vi "Hindbrain Main.vi"(8 "Boat Type":T1, 9 "XBee Serial Port":refnum<visa-resource-name>="LPT1", 11 "NotifierReff":T5) -> ()   [LabVIEW 2013]
doc: "Place to hold all the hindbrain code."
uses:
  Data/TypeDefs/Notifiers.ctl
  Data/TypeDefs/UTM Location.ctl
  Data/TypeDefs/Sail Set Suggestions.ctl
  Data/TypeDefs/Rudder Set Suggestions.ctl
  Data/TypeDefs/OverrideInformation.ctl
  Data/TypeDefs/OverrideMode.ctl
  Data/TypeDefs/MotorSetup.ctl
  Data/TypeDefs/DynamixelSetupInfo.ctl
  Data/TypeDefs/AirmarStatus.ctl
  Data/TypeDefs/HardwareOnline.ctl
  Data/TypeDefs/DynamixelCycleTracker.ctl
  Data/TypeDefs/RC Input Values.ctl
  Classes/Waypoint/Waypoint.lvclass
  Data/TypeDefs/BoatType.ctl
  <vilib>/myRIO/Common/Instrument Driver Framework/myRIO v1.0/UART/vis/myRIO v1.0 Close UART.vi
  <vilib>/myRIO/Common/Instrument Driver Framework/Utilities/vis/FPGA Ref Manager.vi
  <vilib>/myRIO/Common/Instrument Driver Framework/myRIO v1.0/myRIO v1.0 Reset FPGA.vi
  <vilib>/myRIO/Instrument Drivers/Utilities/Utilities.lvlib
  <instrlib>/Dynamixel Motor/Dynamixel Motor.lvlib
panel:
  in  "Tab Control":T2(tab)
  out "Write loop\ncounter":i32
  out "Commanded rudder value":T3 min=-0.95 max=0.95 scale=1.0..-1.0
  out "Commanded sail value":dbl
  out "Dynamixel\nPositions (deg)":dbl[](array[numeric])
  in  "Read actions per\nwrite action":i32=4
  out "Think Counter":i32
  out "Think Heartbeat":bool
  out "Sense Counter":i32
  out "Sense Heartbeat":bool
  out "Act Heartbeat":bool
  out "Read loop counter":i32
  out "Updated Dynamixel Cycles":T4
  in  "Motors Enabled":bool[](array[boolean])=[TRUE, TRUE, TRUE]
  out "Hemisphere Counter":i32
  out "Airmar Counter":i32
  out "Hemi Compass":dbl
  out "Airmar Compass":dbl
  out "String written to XBee":string
  out "String received from XBee":string
  out "UDP Time Out?":bool
  out "Battery Volts":dbl
  out "Replace? (<6?)":bool
  in  "Wind Speed":dbl
  out "XBee Sense/Act Counter":i32
  out "XBee Sense/Act Heartbeat":bool
  out "Camera Sense Counter":i32
  out "Camera Sense Heartbeat":bool
  out "Think Counter":i32
  out "Think Heartbeat":bool
  # "Timing"
  # "Timing"
  # "If you're getting no strings, do you have the right COM port?"
  # "Camera"
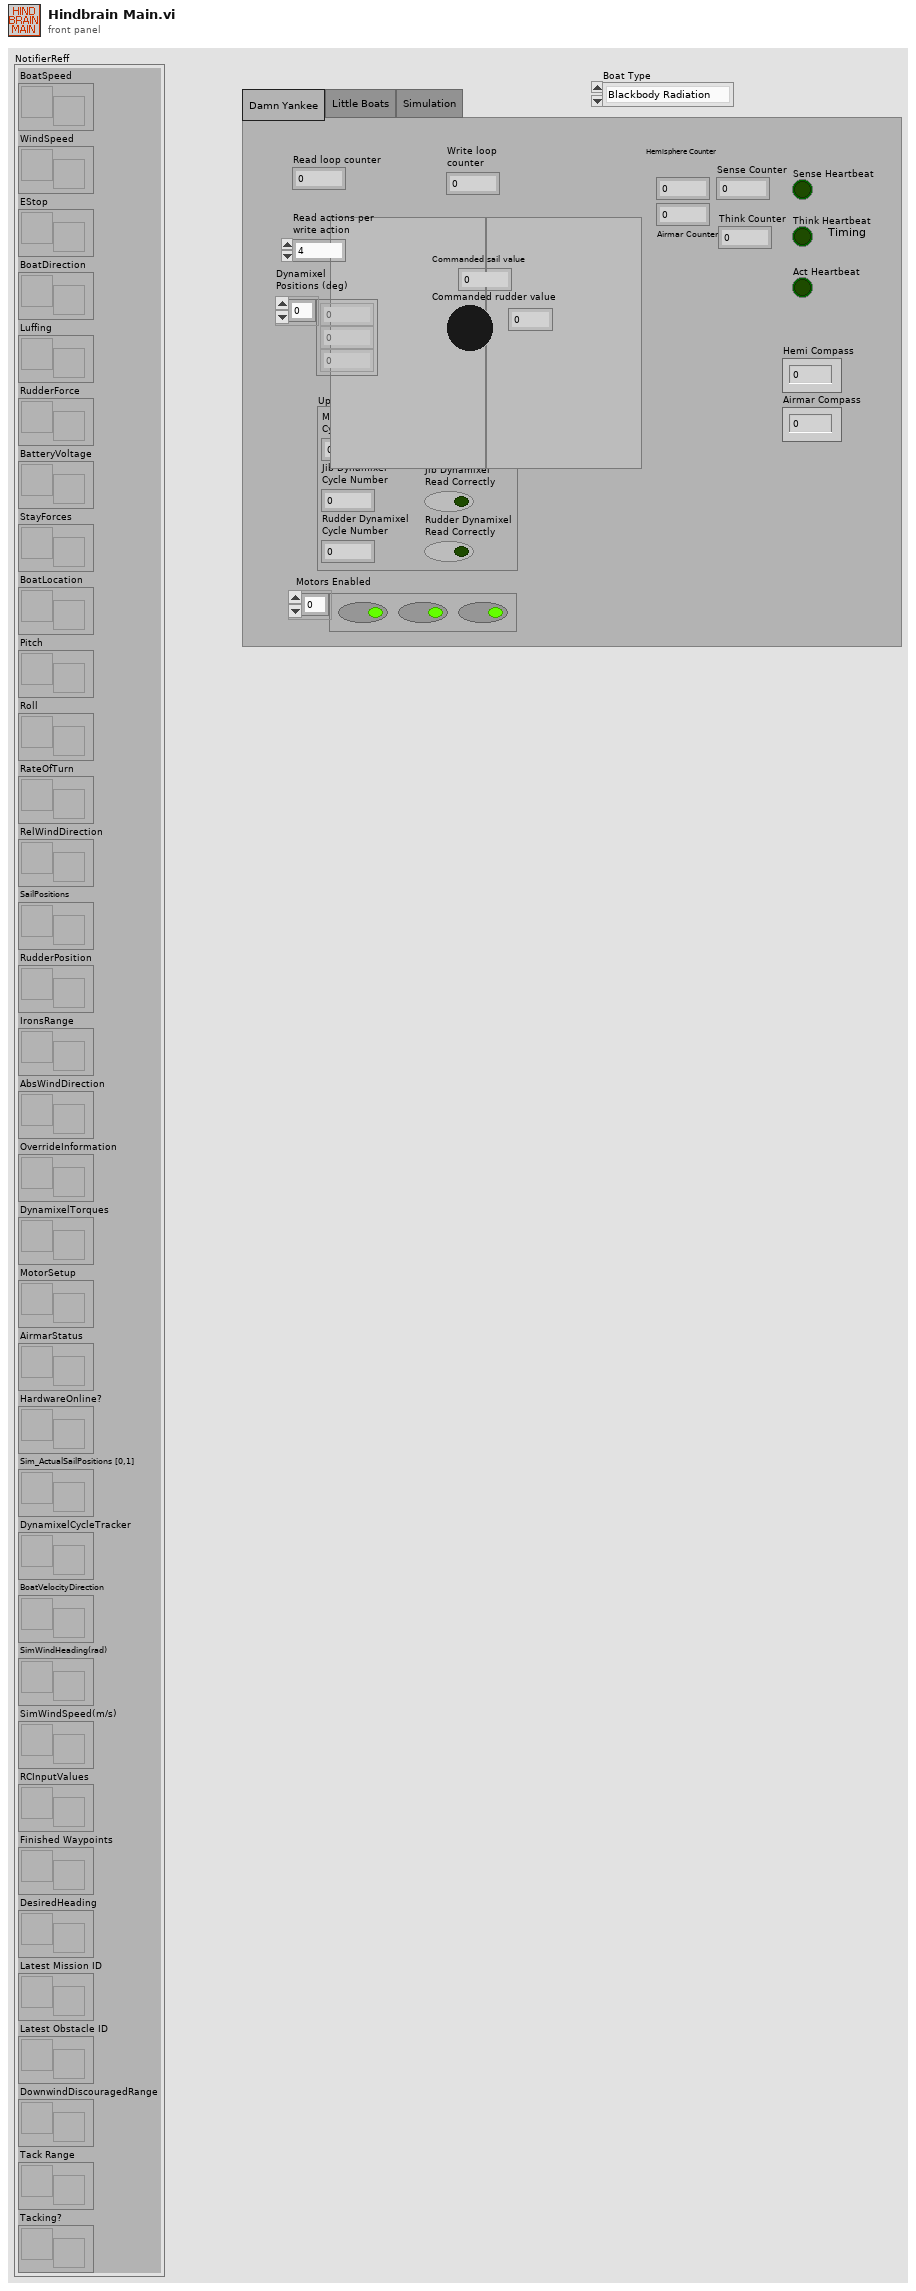
[diagram p1: front panel]
types:
  T1 = typedef "BoatType.ctl" = enum16{"Blackbody Radiation", "ReadLog", "Little boats", "Damn Yankee"}
  T2 = enum32{"Damn Yankee", "Little Boats", "Simulation"}
  T3 = typedef "Rudder Set Suggestions.ctl" = dbl
  T4 = typedef "DynamixelCycleTracker.ctl" = cluster{"Main Dynamixel\nCycle Number":i32, "Jib Dynamixel\nCycle Number":i32, "Rudder Dynamixel\nCycle Number":i32, "Main Dynamixel\nRead Correctly":bool, "Jib Dynamixel\nRead Correctly":bool, "Rudder Dynamixel\nRead Correctly":bool}
  T5 = typedef "Notifiers.ctl" = cluster{"BoatSpeed":refnum<notifier>, "WindSpeed":refnum<notifier>, "EStop":refnum<notifier>, "BoatDirection":refnum<notifier>, "Luffing":refnum<notifier>, "RudderForce":refnum<notifier>, "BatteryVoltage":refnum<notifier>, "StayForces":refnum<notifier>, "BoatLocation":refnum<notifier>, "Pitch":refnum<notifier>, "Roll":refnum<notifier>, "RateOfTurn":refnum<notifier>, "RelWindDirection":refnum<notifier>, "SailPositions":refnum<notifier>, "RudderPosition":refnum<notifier>, "IronsRange":refnum<notifier>, "AbsWindDirection":refnum<notifier>, "OverrideInformation":refnum<notifier>, "DynamixelTorques":refnum<notifier>, "MotorSetup":refnum<notifier>, "AirmarStatus":refnum<notifier>, "HardwareOnline?":refnum<notifier>, "Sim_ActualSailPositions [0,1]":refnum<notifier>, "DynamixelCycleTracker":refnum<notifier>, "BoatVelocityDirection":refnum<notifier>, "SimWindHeading(rad)":refnum<notifier>, "SimWindSpeed(m/s)":refnum<notifier>, "RCInputValues":refnum<notifier>, "Finished Waypoints":refnum<notifier>, "DesiredHeading":refnum<notifier>, "Latest Mission ID":refnum<notifier>, "Latest Obstacle ID":refnum<notifier>, "DownwindDiscouragedRange":refnum<notifier>, "Tack Range":refnum<notifier>, "Tacking?":refnum<notifier>}
  T6 = typedef "GPS-Compass Queue Cluster.ctl" = cluster{"BoatLocation Queue":refnum<queue>, "BoatDirection Queue":refnum<queue>, "BoatSpeed Queue":refnum<queue>, "RateOfTurn Queue":refnum<queue>, "Pitch Queue":refnum<queue>, "Roll Queue":refnum<queue>, "BoatVelocityDirection Queue ":refnum<queue>}
  T7 = typedef "WindData Queue Cluster.ctl" = cluster{"RelWindDirection Queue":refnum<queue>, "WindSpeed Queue":refnum<queue>, "AbsWindDirection Queue":refnum<queue>}
  T8 = cluster{"Shroud Queue":refnum<queue>, "Battery Voltage Queue":refnum<queue>, "Accelerometer Queue":refnum<queue>, "AirmarGPS-Compass Queue Cluster":T6, "Hemisphere Queue Cluster":T6, "Airmar Wind Queue Cluster":T7, "Wind Vane Queue Cluster":T7, "Little Boat Queues":cluster{"Heading Queue":refnum<queue>, "Location Queue":refnum<queue>, "Wind Speed Queue":refnum<queue>, "Tilt Queue":refnum<queue>, "Wind Direction Queue":refnum<queue>}, "DynamixelTorque Queue":refnum<queue>, "DynamixelPosition Queue":refnum<queue>}
  T9 = typedef "MotorSetup.ctl" = cluster{"Main Dynamixel Set Data":T10, "Rudder Dynamixel Set Data":T10, "Jib Dynamixel Set Data":T10}
  T10 = typedef "DynamixelSetupInfo.ctl" = cluster{"Lower Winch Bound (deg)":dbl, "Upper Winch Bound (deg)":dbl}
  T11 = typedef "DamnYankeeIOPorts.ctl" = cluster{"Airmar VISA Resource":refnum<visa-resource-name>, "Hemisphere VISA Resource":refnum<visa-resource-name>, "Dynamixel VISA Resource":refnum<visa-resource-name>, "Airmar Error":errorcluster, "Hemisphere Error":errorcluster, "Dynamixel Error":errorcluster, "FPGA Error":errorcluster, "FPGA VI Reference Out":refnum<k20>, "Motors IDs Found":u8[]}
  T12 = cluster{"Heading Queue":refnum<queue>, "Location Queue":refnum<queue>, "Wind Speed Queue":refnum<queue>, "Tilt Queue":refnum<queue>, "Wind Direction Queue":refnum<queue>}
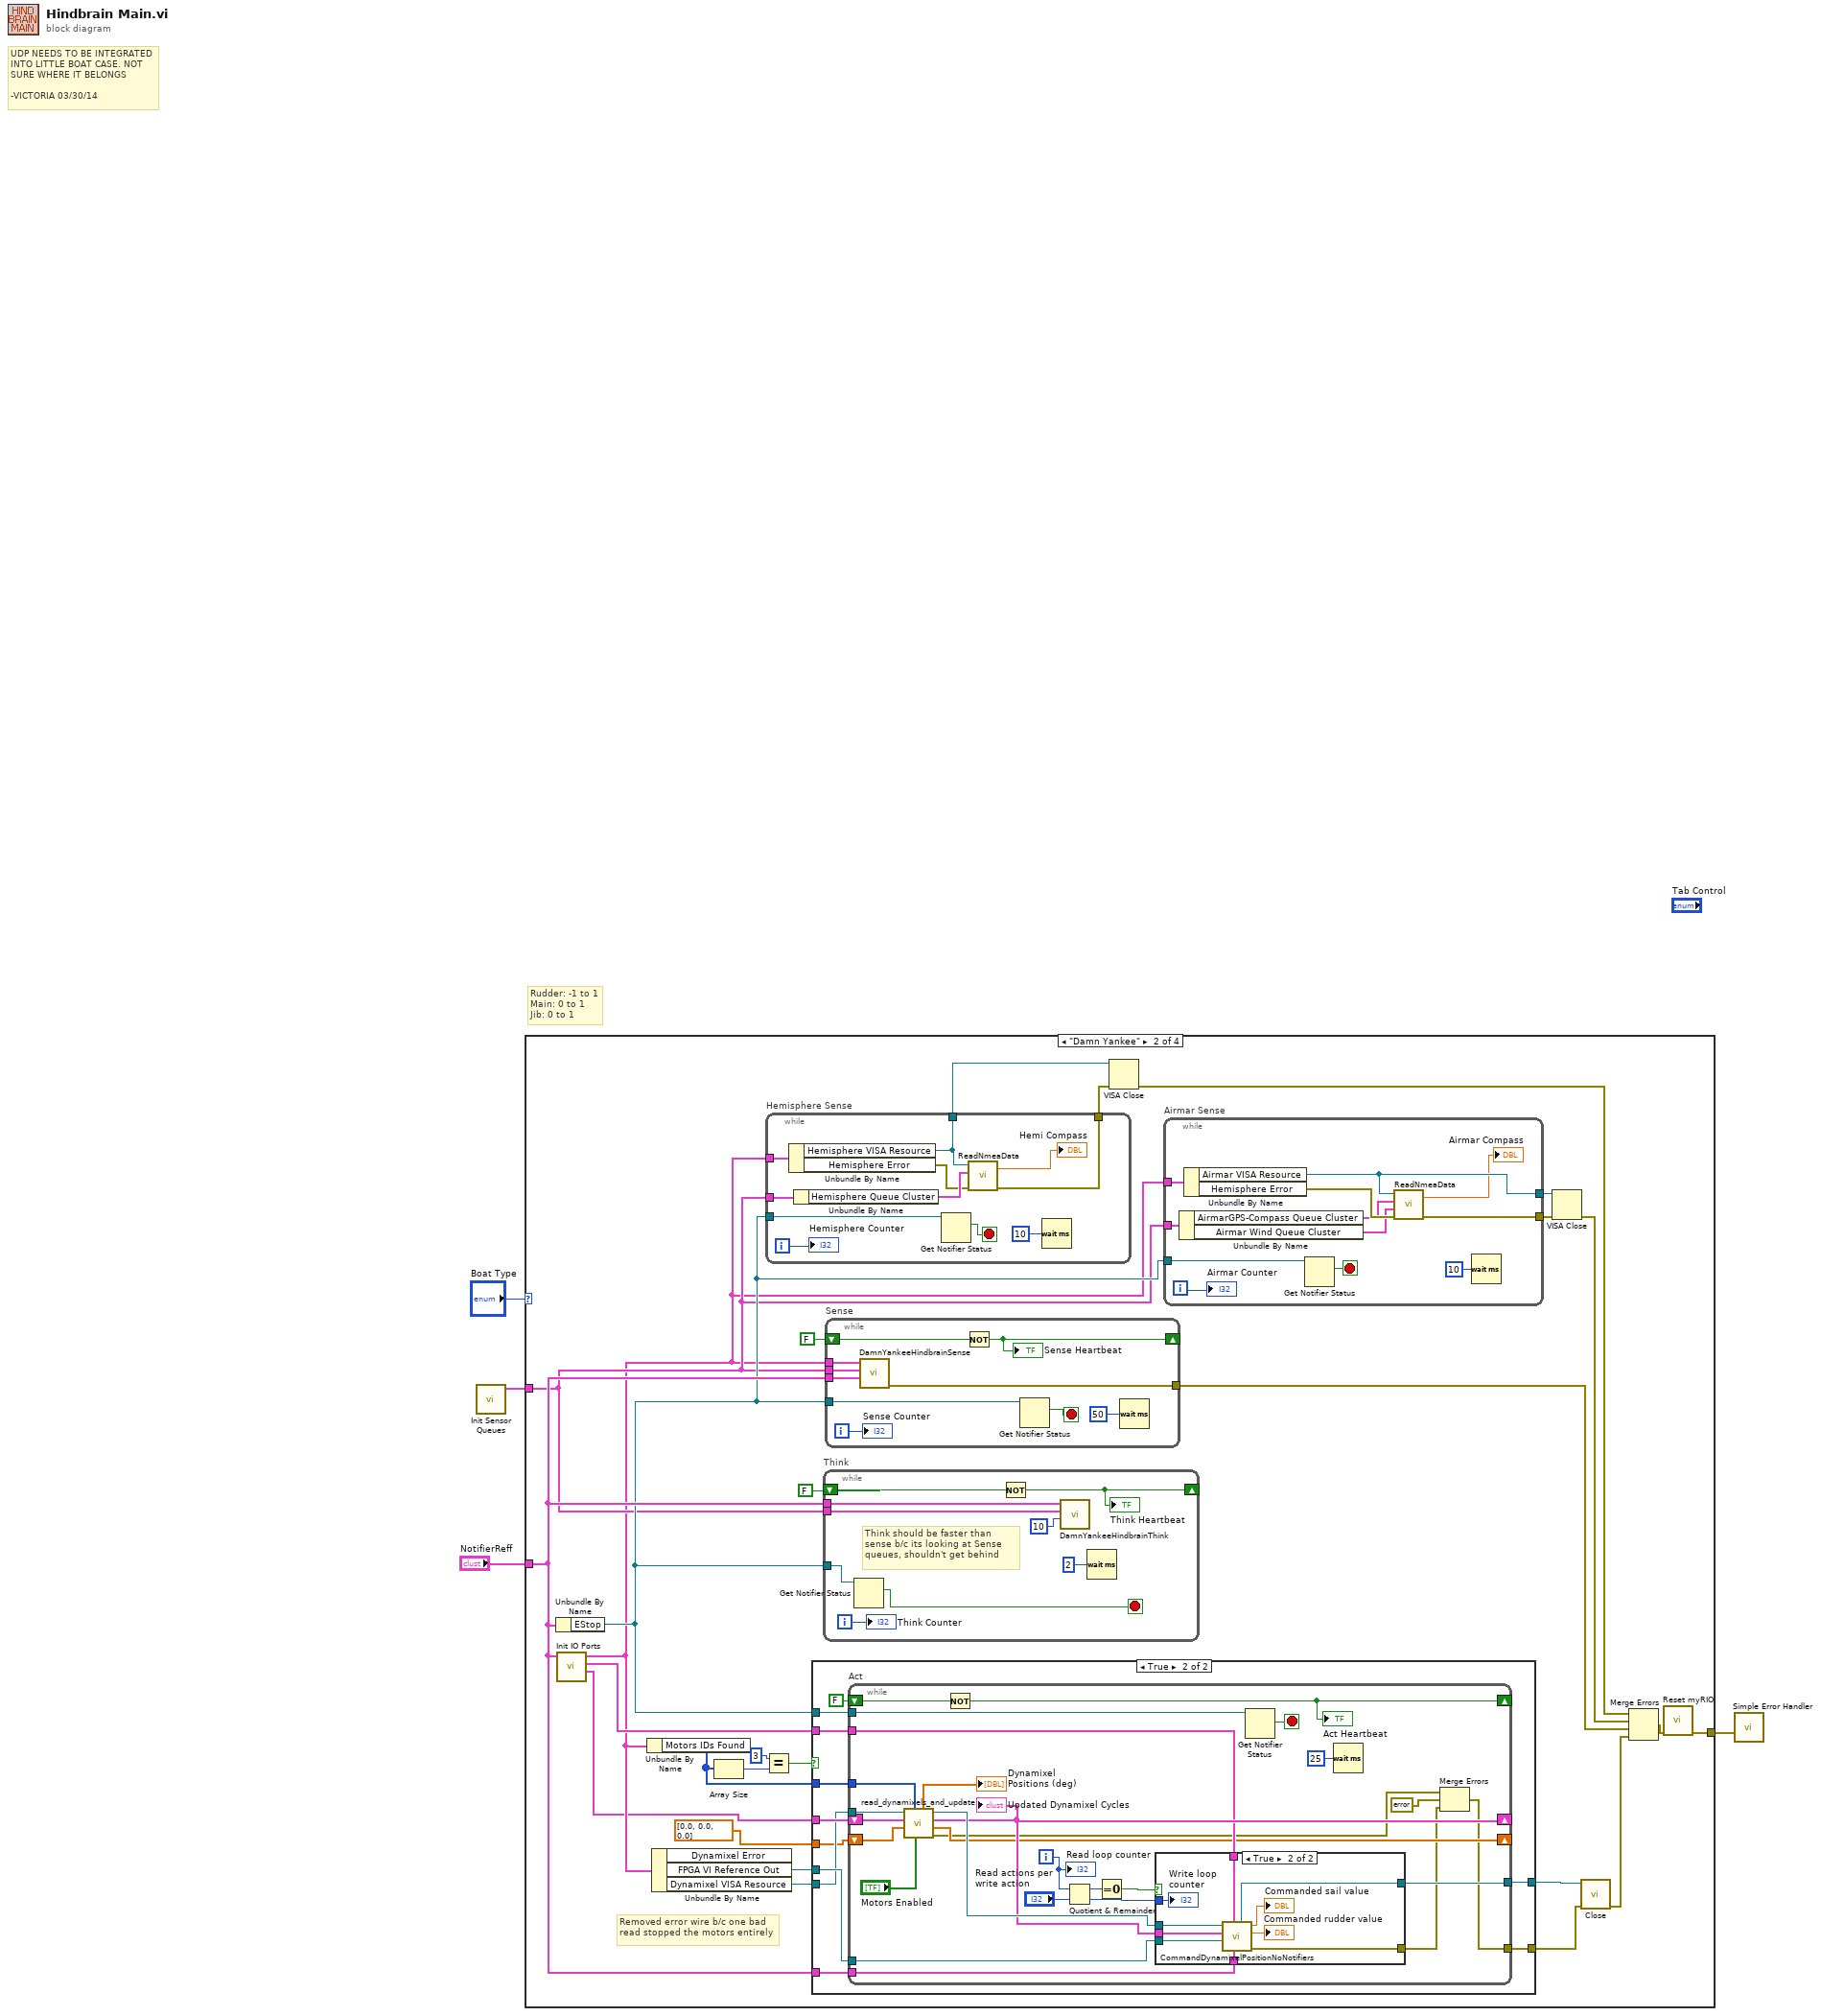
[diagram p0: block diagram]
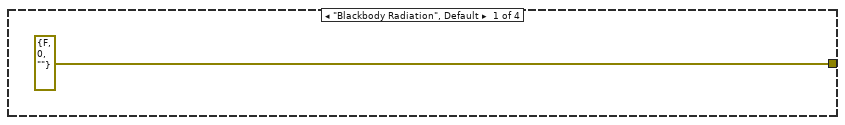
[diagram p2: hidden frame]
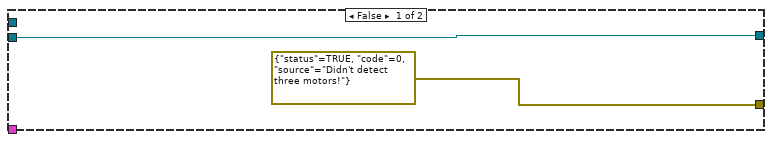
[diagram p3: hidden frame]
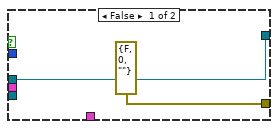
[diagram p4: hidden frame]
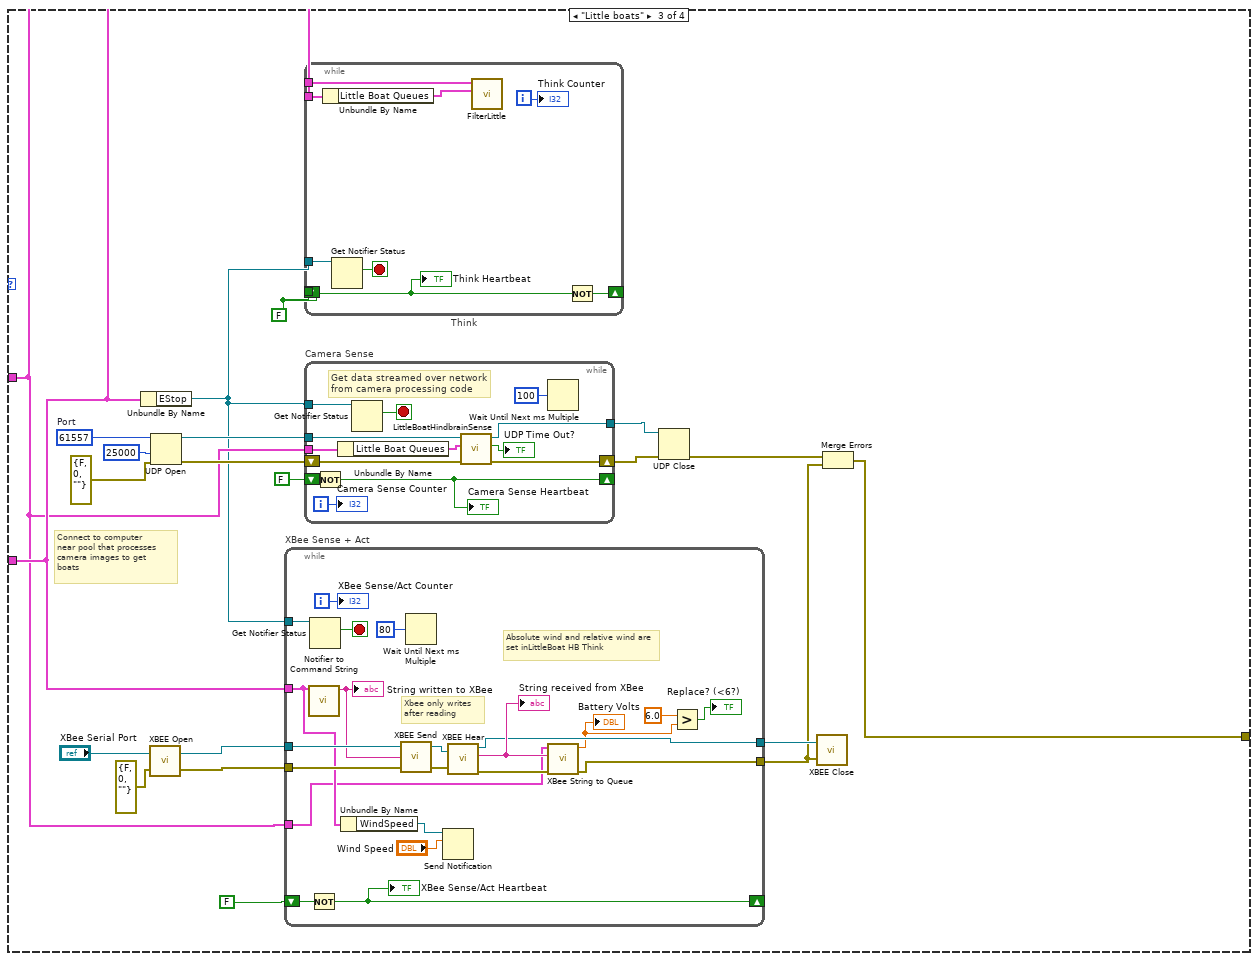
[diagram p5: hidden frame]
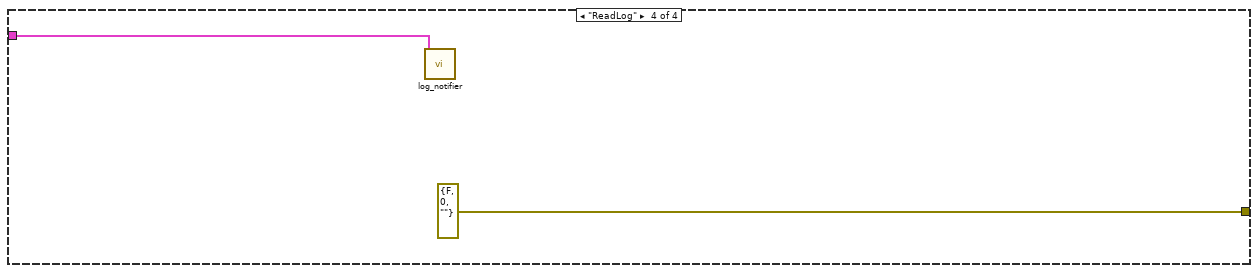
[diagram p6: hidden frame]
diagram:
  # "Rudder: -1 to 1\nMain: 0 to 1 \nJib: 0 to 1"
  # "UDP NEEDS TO BE INTEGRATED\nINTO LITTLE BOAT CASE. NOT \nSURE WHERE IT BELONGS\n\n-VICTORIA 03/30/14"
  n1 = call "Init Sensor Queues.vi"() -> ("output cluster"=w4:T8)  [unwired: 11 in]
  n2 = case shown="\"Damn Yankee\"" "Boat Type" {
    tunnel: w4 -> [_ w15 w136 _]
    tunnel: "NotifierReff" -> [_ w18 w140 w191]
    tunnel: [errorcluster {"status"=FALSE, "code"=0, "source"=""} ("error IO") w31 w147 errorcluster {"status"=FALSE, "code"=0, "source"=""} ("error IO")] -> w3
    frame "Blackbody Radiation", Default {
    }
    frame "Damn Yankee" {
      # "Removed error wire b/c one bad read stopped the motors entirely"
      n3 = Unbundle By Name(w18) -> ("EStop"=w16:refnum<notifier>)
      n4 = call "Init IO Ports.vi"("NotifierReff"=w18) -> ("Dynamixel Cycles"=w6:T4, "Dynamixel Bounds Out"=w23:T9, "IO Port Cluster"=w14:T11)  [unwired: 8 in]
      n5 = Unbundle By Name(w14) -> ("Motors IDs Found"=w24:u8[])
      n6 = Unbundle By Name(w14) -> ("FPGA VI Reference Out"=w25:refnum<k20>, "Dynamixel VISA Resource"=w22:refnum<visa-resource-name>)  [unwired: 1 out]
      n7 = Array Size(array=w24) -> (size(s)=w28:i32)
      n8 = Equal?(x=3, y=w28) -> (x = y?=w27:bool)
      n9 = while "Hemisphere Sense" {
        tunnel: w14 -> [w55]
        tunnel: w15 -> [w54]
        tunnel: w16 -> [w50]
        tunnel: [w48] -> w13
        tunnel: [w47] -> w12
        i -> [w51]
        stop <- w49 stop-if-true
        n10 = Unbundle By Name(w55) -> ("Hemisphere VISA Resource"=w48:refnum<visa-resource-name>, "Hemisphere Error"=w52:errorcluster)
        n11 = Unbundle By Name(w54) -> ("Hemisphere Queue Cluster"=w53:T6)
        n12 = Get Notifier Status(notifier=w50) -> (current notification=w49:bool)  [unwired: 1 in, 4 out]
        n13 = call "ReadNmeaData.vi"("error in"=w52, "GPS-Compass Queue Cluster"=w53, "Serial Port"=w48) -> ("error out"=w47:errorcluster, "Boat Direction 2"=→"Hemi Compass":dbl)  [unwired: 2 in, 5 out]
        n14 = Wait (ms)(milliseconds to wait=u32 10) -> ()  [unwired: 1 out]
        "Hemisphere Counter" <- w51
      }
      n15 = case shown="True" w27 {
        tunnel: [errorcluster {"status"=TRUE, "code"=0, "source"="Didn't detect three motors!"} ("error out") w58] -> w20
        tunnel: w16 -> [_ w67]
        tunnel: w23 -> [_ w66]
        tunnel: w6 -> [_ w65]
        tunnel: [w56 w64] -> w21
        tunnel: w25 -> [_ w63]
        tunnel: w24 -> [_ w62]
        tunnel: w22 -> [w56 w61]
        tunnel: w18 -> [_ w60]
        tunnel: dbl[] [0.0, 0.0, 0.0] -> [_ w59]
        frame False {
        }
        frame True {
          n16 = while "Act" {
            tunnel: w66 -> [w81]
            tunnel: w67 -> [w94]
            shift-right: [w93] -> _
            shift-left: FALSE -> [w92]
            shift-right: [w82] -> _
            shift-left: w65 -> [w83]
            tunnel: [w80] -> w64
            shift-right: [w79] -> _
            shift-left: w59 -> [w78]
            tunnel: w63 -> [w75]
            tunnel: w62 -> [w74]
            tunnel: w61 -> [w72]
            tunnel: w60 -> [w71]
            tunnel: [w69] -> w58
            i -> [w73]
            stop <- w95 stop-if-true
            n17 = call "read_dynamixels_and_update.vi"("Motors Enabled"="Motors Enabled", "Motors IDs Found"=w74, "Last read positions"=w78, "Dynamixel Cycle Constant"=w83, "VISA Refnum in"=w72) -> ("error out"=w77:errorcluster[], "Latest read positions (dyn)"=w79:dbl[], "Updated Dynamixle Cycles"=w82:T4, "VISA Refnum out"=w89:refnum<visa-resource-name>, "Dynamixel\nPositions (deg)"=→"Dynamixel\nPositions (deg)":dbl[])  [unwired: 2 in]
            "Updated Dynamixel Cycles" <- w82
            n18 = Not(x=w92) -> (.not. x?=w93:bool)
            "Act Heartbeat" <- w93
            n19 = Quotient & Remainder(x=w73, y="Read actions per\nwrite action") -> (x-y*floor(x/y)=w87:i32, floor(x/y)=w85:i32)
            n20 = Equal To 0?(x=w87) -> (x = 0?=w86:bool)
            n21 = case shown="True" w86 {
              tunnel: w75 -> [_ w107]
              tunnel: w81 -> [_ w99]
              tunnel: w89 -> [w97 w106]
              tunnel: w82 -> [_ w105]
              tunnel: [errorcluster {"status"=FALSE, "code"=0, "source"=""} ("Error out") w102] -> w70
              tunnel: [w97 w101] -> w80
              tunnel: w85 -> [_ w100]
              tunnel: w71 -> [_ w98]
              frame False {
              }
              frame True {
                n22 = call "CommandDynamixelPositionNoNotifiers.vi"("NotifierReff"=w98, "Dynamixel Bounds"=w99, "FPGA VI Reference In"=w107, "Dynamixel Cycles"=w105, "VISA resource name"=w106) -> ("Error out"=w102:errorcluster, "Commanded rudder value"=→"Commanded rudder value":T3, "Debug sail value"=→"Commanded sail value":dbl, "VISA resource name OUT"=w101:refnum<visa-resource-name>)  [unwired: 3 in]
                "Write loop\ncounter" <- w100
              }
            }
            n23 = Get Notifier Status(notifier=w94) -> (current notification=w95:bool)  [unwired: 1 in, 4 out]
            n24 = Wait (ms)(milliseconds to wait=u32 25) -> ()  [unwired: 1 out]
            n25 = Merge Errors(w77, errorcluster {"status"=FALSE, "code"=0, "source"=""} ("error IO"), w70) -> (w69:errorcluster)
            "Read loop counter" <- w73
          }
        }
      }
      n26 = while "Think" {
        tunnel: w16 -> [w116]
        tunnel: w15 -> [w110]
        tunnel: w18 -> [w114]
        shift-right: [w111] -> _
        shift-left: FALSE -> [w112]
        i -> [w113]
        stop <- w115 stop-if-true
        # "Think should be faster than sense b/c its looking at Sense queues, shouldn't get behind"
        n27 = Get Notifier Status(notifier=w116) -> (current notification=w115:bool)  [unwired: 1 in, 4 out]
        n28 = Not(x=w112) -> (.not. x?=w111:bool)
        "Think Heartbeat" <- w111
        n29 = call "DamnYankeeHindbrainThink.vi"("Queue timeout (ms)"=10, "Data queue cluster"=w110, "Notifier References"=w114) -> ()  [unwired: 9 in]
        n30 = Wait (ms)(milliseconds to wait=u32 2) -> ()  [unwired: 1 out]
        "Think Counter" <- w113
      }
      n31 = while "Sense" {
        tunnel: w14 -> [w118]
        tunnel: w18 -> [w126]
        tunnel: w15 -> [w122]
        tunnel: [w125] -> w7
        tunnel: w16 -> [w124]
        shift-right: [w119] -> _
        shift-left: FALSE -> [w120]
        i -> [w121]
        stop <- w123 stop-if-true
        n32 = call "DamnYankeeHindbrainSense.vi"("Notifier References"=w126, "Data Queue clusters"=w122, "IO Cluster"=w118) -> ("error out"=w125:errorcluster)  [unwired: 8 in]
        n33 = Not(x=w120) -> (.not. x?=w119:bool)
        "Sense Heartbeat" <- w119
        n34 = Get Notifier Status(notifier=w124) -> (current notification=w123:bool)  [unwired: 1 in, 4 out]
        n35 = Wait (ms)(milliseconds to wait=u32 50) -> ()  [unwired: 1 out]
        "Sense Counter" <- w121
      }
      n36 = VISA Close(VISA resource name=w13, error in (no error)=w12) -> (error out=w10:errorcluster)
      n37 = while "Airmar Sense" {
        tunnel: w14 -> [w44]
        tunnel: w15 -> [w43]
        tunnel: w16 -> [w41]
        tunnel: [w39] -> w11
        tunnel: [w34] -> w8
        i -> [w42]
        stop <- w40 stop-if-true
        n38 = Unbundle By Name(w43) -> ("AirmarGPS-Compass Queue Cluster"=w36:T6, "Airmar Wind Queue Cluster"=w37:T7)
        n39 = Unbundle By Name(w44) -> ("Airmar VISA Resource"=w34:refnum<visa-resource-name>, "Hemisphere Error"=w38:errorcluster)
        n40 = Get Notifier Status(notifier=w41) -> (current notification=w40:bool)  [unwired: 1 in, 4 out]
        n41 = call "ReadNmeaData.vi"("error in"=w38, "Airmar Wind Queue Cluster"=w37, "GPS-Compass Queue Cluster"=w36, "Serial Port"=w34) -> ("error out"=w39:errorcluster, "Boat Direction 2"=→"Airmar Compass":dbl)  [unwired: 1 in, 5 out]
        n42 = Wait (ms)(milliseconds to wait=u32 10) -> ()  [unwired: 1 out]
        "Airmar Counter" <- w42
      }
      n43 = VISA Close(VISA resource name=w8, error in (no error)=w11) -> (error out=w9:errorcluster)
      n44 = call <instrlib>:"Close.vi"("error in (no error)"=w20, "VISA resource name"=w21) -> ("error out"=w19:errorcluster)  [unwired: 9 in]
      n45 = Merge Errors "Merge Errors"(w10, w9, w7, w19) -> (w32:errorcluster)
      n46 = call <vilib>:"Reset myRIO.vi"("error in (no error)"=w32) -> ("error out"=w31:errorcluster)  [unwired: 10 in]
    }
    frame "Little boats" {
      w127 = FALSE
      w145 = u16 61557  # Port
      # "Connect to computer\nnear pool that processes\ncamera images to get\nboats"
      n47 = Unbundle By Name(w140) -> ("EStop"=w130:refnum<notifier>)
      n48 = call "XBEE Open.vi"("error in"=errorcluster {"status"=FALSE, "code"=0, "source"=""}, "VISA resource name"="XBee Serial Port") -> ("error out"=w139:errorcluster, "VISA resource name out"=w141:refnum<visa-resource-name>)
      n49 = UDP Open(8:errorcluster {"status"=FALSE, "code"=0, "source"=""} ("error in (no error)"), 9:25000 ("timeout ms (25000)"), 11:w145) -> (port=w138:refnum<k16>, 0:w137:errorcluster)  [unwired: 2 in, 1 out]
      n50 = while "XBee Sense + Act" {
        tunnel: w141 -> [w181]
        tunnel: w140 -> [w167]
        tunnel: w130 -> [w182]
        tunnel: w136 -> [w162]
        tunnel: [w172] -> w135
        tunnel: w139 -> [w180]
        tunnel: [w171] -> w134
        shift-right: [w164] -> _
        shift-left: FALSE -> [w165]
        i -> [w163]
        stop <- w176 stop-if-true
        # "Absolute wind and relative wind are set inLittleBoat HB Think"
        # "Xbee only writes\nafter reading"
        n51 = call "Notifier to Command String.vi"("NotifierReff"=w167) -> ("String"=w179:string)  [unwired: 10 in]
        "String written to XBee" <- w179
        n52 = Not(x=w165) -> (.not. x?=w164:bool)
        "XBee Sense/Act Heartbeat" <- w164
        n53 = Get Notifier Status(notifier=w182) -> (current notification=w176:bool)  [unwired: 1 in, 4 out]
        n54 = Unbundle By Name(w167) -> ("WindSpeed"=w166:refnum<notifier>)
        n55 = call "XBEE Send.vi"("error in (no error)"=w180, "String"=w179, "VISA resource name"=w181) -> ("error out"=w177:errorcluster, "VISA resource name out"=w178:refnum<visa-resource-name>)  [unwired: 1 out]
        n56 = Wait Until Next ms Multiple(millisecond multiple=u32 80) -> ()  [unwired: 1 out]
        n57 = Send Notification(notification="Wind Speed", notifier=w166) -> ()  [unwired: 1 in, 2 out]
        n58 = call "XBEE Hear.vi"("VISA resource name"=w178, "error in (no error)"=w177) -> ("VISA resource name out"=w172:refnum<visa-resource-name>, "String Received"=w175:string, "error out"=w174:errorcluster)  [unwired: 1 out]
        "String received from XBee" <- w175
        n59 = call "XBee String to Queue.vi"("error in (no error)"=w174, "String Received"=w175, "Queue cluster"=w162) -> ("error out"=w171:errorcluster, "Battery Volts"=w170:dbl)  [unwired: 7 in]
        "Battery Volts" <- w170
        n60 = Greater?(x=6.0, y=w170) -> (0:→"Replace? (<6?)":bool)
        "XBee Sense/Act Counter" <- w163
      }
      n61 = while "Think" {
        tunnel: w130 -> [w190]
        tunnel: w136 -> [w188]
        tunnel: w140 -> [w186]
        shift-right: [w184] -> _
        shift-left: w127 -> [w183]
        tunnel: w127 -> [_]
        i -> [w185]
        stop <- w189 stop-if-true
        n62 = Unbundle By Name(w188) -> ("Little Boat Queues"=w187:T12)
        n63 = Get Notifier Status(notifier=w190) -> (current notification=w189:bool)  [unwired: 1 in, 4 out]
        n64 = call "FilterLittle.vi"("Little Boat Queues"=w187, "NotifierReff"=w186) -> ()  [unwired: 10 in]
        n65 = Not(x=w183) -> (.not. x?=w184:bool)
        "Think Counter" <- w185
        "Think Heartbeat" <- w183
      }
      n66 = while "Camera Sense" {
        tunnel: w138 -> [w159]
        tunnel: w136 -> [w158]
        tunnel: [w156] -> w133
        tunnel: w130 -> [w153]
        shift-right: [w155] -> w132
        shift-left: w137 -> [w160]
        shift-right: [w148] -> _
        shift-left: FALSE -> [w149]
        i -> [w150]
        stop <- w152 stop-if-true
        # "Get data streamed over network from camera processing code"
        n67 = Not(x=w149) -> (.not. x?=w148:bool)
        "Camera Sense Heartbeat" <- w148
        n68 = Unbundle By Name(w158) -> ("Little Boat Queues"=w157:T12)
        n69 = Get Notifier Status(notifier=w153) -> (current notification=w152:bool)  [unwired: 1 in, 4 out]
        n70 = call "LittleBoatHindbrainSense.vi"("error in (no error)"=w160, "Little Boat Queues"=w157, "connection ID"=w159) -> ("error out"=w155:errorcluster, "UDP Time Out?"=→"UDP Time Out?":bool, "connection ID out"=w156:refnum<k16>)  [unwired: 6 in]
        n71 = Wait Until Next ms Multiple(millisecond multiple=u32 100) -> ()  [unwired: 1 out]
        "Camera Sense Counter" <- w150
      }
      n72 = UDP Close(connection ID=w133, 8:w132) -> (error out=w131:errorcluster)  [unwired: 1 out]
      n73 = call "XBEE Close.vi"("error in (no error)"=w134, "VISA resource name"=w135) -> ()
      n74 = Merge Errors "Merge Errors"(w131, w134) -> (w147:errorcluster)
    }
    frame "ReadLog" {
      n75 = call "log_notifier.vi"("NotifierReferences"=w191) -> ()  [unwired: 11 in]
    }
  }
  n76 = call <vilib>:"Simple Error Handler.vi"("error in (no error)"=w3) -> ()  [unwired: 4 in, 5 out]
